vi "Update Logger State.vi"(8 "error in (no error)":errorcluster, 10 "Logger State":T1, 11 "Module in":refnum<class "Module.lvclass">) -> (0 "error out":errorcluster, 3 "Module":refnum<class "Module.lvclass">)   [LabVIEW 2020, in "VolatusData.lvlib"]
uses:
  VolatusData.lvlib
  Volatus/Module/Module.lvclass
  Logger State.ctl
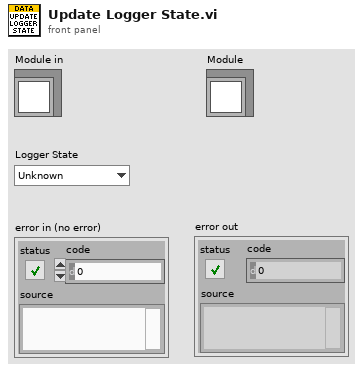
[diagram p1: front panel]
types:
  T1 = typedef "VolatusData.lvlib/Logger State.ctl" = enum16{"Unknown", "Idle", "Preparing", "Ready", "Logging", "Stopping"}
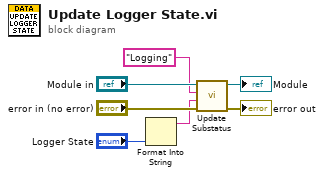
[diagram p0: block diagram]
diagram:
  n1 = Format Into String("Logger State") -> (resulting string=w2:string)  [unwired: 3 in, 1 out]
  n2 = call "Update Substatus.vi"("error in (no error)"="error in (no error)", "Status"=w2, "Name"="Logging", "Module in"="Module in") -> ("error out"=→"error out":errorcluster, "Module out"=→"Module":refnum<class "Module.lvclass">)  [unwired: 6 in]
